vi "Set Digitals (Batch).vi"(0 "connection ID":refnum<k16>, 1 "address":u32, 2 "port":u16, 5 "Mask":bool[](array[boolean])=[TRUE, TRUE, TRUE, TRUE, TRUE, TRUE, TRUE, TRUE, TRUE, TRUE, TRUE, TRUE, TRUE, TRUE, TRUE, TRUE], 7 "Digital State":T1 items=["LOW", "HIGH"], 9 "timeout ms (1000)":i32=1000, 11 "error in (no error)":errorcluster) -> (4 "connection ID out":refnum<k16>, 6 "received data":string, 15 "error out":errorcluster)   [LabVIEW 2016, in "instr.lvlib"]
doc: "Sets all digitals to a given state. Batch operation. This affects the digital IO mode as necessary."
uses:
  instr.lvlib
  IO State.ctl
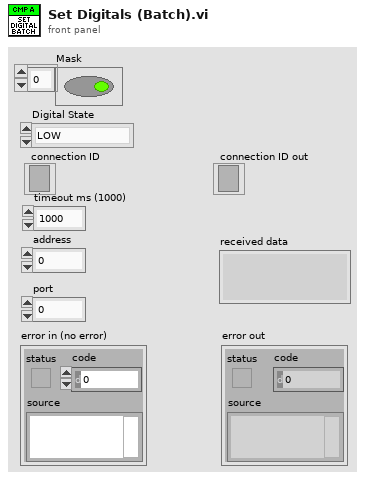
[diagram p1: front panel]
types:
  T1 = typedef "instr.lvlib/IO State.ctl" = u16
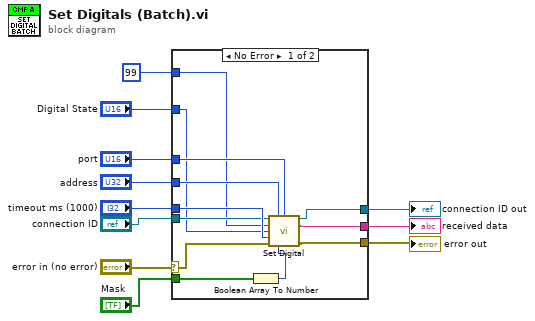
[diagram p0: block diagram]
diagram:
  n1 = case shown="No Error" "error in (no error)" {
    selector: "error in (no error)" -> [w23 w25]
    tunnel: [w18 w25] -> w11
    tunnel: [w19 _] -> w9
    tunnel: "timeout ms (1000)" -> [w22 _]
    tunnel: "connection ID" -> [w21 w24]
    tunnel: [w20 w24] -> w6
    tunnel: u16 99 ("Digital Number") -> [w14 _]
    tunnel: "Digital State" -> [w15 _]
    tunnel: "address" -> [w16 _]
    tunnel: "port" -> [w17 _]
    tunnel: "Mask" -> [w12 _]
    frame No Error {
      n2 = Boolean Array To Number(Boolean array=w12) -> (number=w13:u32)
      n3 = call "Set Digital.vi"("connection ID"=w21, "address"=w16, "port"=w17, "Digital Number"=w14, "Digital State"=w15, "timeout ms (1000)"=w22, "error in (no error)"=w23, "mask"=w13) -> ("connection ID out"=w20:refnum<k16>, "received data"=w19:string, "error out"=w18:errorcluster)  [unwired: 5 in]
    }
    frame Error {
    }
  }
  "error out" <- w11
  "received data" <- w9
  "connection ID out" <- w6
